vi "set_plot_lc.vi"(4 "lc_scale_settings":enum32{"autoscale", "fancy_scale", "zero_scale"}(ring), 6 "plot_lc_ref":refnum<vi>, 7 "set_scale":bool, 8 "enable_plot_lp":bool, 9 "enable_plot_ls":bool, 10 "enable_plot_cp":bool, 11 "enable_plot_cs":bool) -> ()   [LabVIEW 2025]
uses:
  82382b49-3e9a-49aa-a7d7-4b7aa8e385a1.vi
  98033bfd-429a-49ec-a4ef-dc58c613fc7d.vi
  0a7f9e3b-32db-4052-a28a-afecad899844.vi
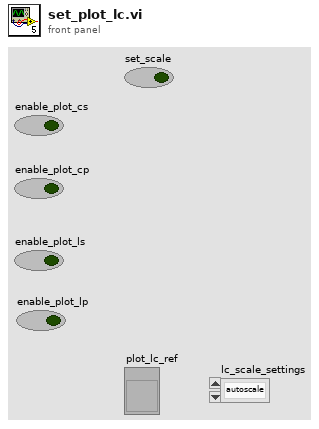
[diagram p1: front panel]
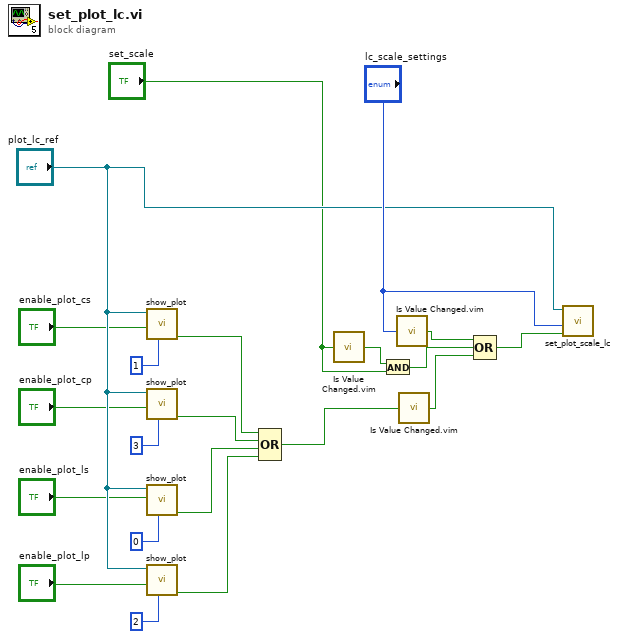
[diagram p0: block diagram]
diagram:
  n1 = call "show_plot.vi"("plot_id"=1 ("y_scale_id"), "show_plot"="enable_plot_cs", "XYGraph Refnum"="plot_lc_ref") -> ("done"=w4:bool)  [unwired: 8 in]
  n2 = call "show_plot.vi"("plot_id"=3 ("y_scale_id"), "show_plot"="enable_plot_cp", "XYGraph Refnum"="plot_lc_ref") -> ("done"=w3:bool)  [unwired: 8 in]
  n3 = call "show_plot.vi"("plot_id"=0 ("y_scale_id"), "show_plot"="enable_plot_ls", "XYGraph Refnum"="plot_lc_ref") -> ("done"=w2:bool)  [unwired: 8 in]
  n4 = call "show_plot.vi"("plot_id"=2 ("y_scale_id"), "show_plot"="enable_plot_lp", "XYGraph Refnum"="plot_lc_ref") -> ("done"=w1:bool)  [unwired: 8 in]
  n5 = Compound Arithmetic op=OR(w4, w3, w2, w1) -> (w5:bool)
  n6 = call "Is Value Changed.vim"("value"="set_scale") -> ("changed or first call?"=w17:bool)
  n7 = And(x=w17, y="set_scale") -> (x .and. y?=w16:bool)
  n8 = call "Is Value Changed.vim"("value"="lc_scale_settings") -> ("changed or first call?"=w19:bool)
  n9 = call "Is Value Changed.vim"("value"=w5) -> ("changed or first call?"=w18:bool)
  n10 = Compound Arithmetic op=OR(w19, w16, w18) -> (w21:bool)
  n11 = call "set_plot_scale_lc.vi"("set_scale"=w21, "lc_scale_settings"="lc_scale_settings", "plot_lc_ref"="plot_lc_ref") -> ()  [unwired: 9 in]
